vi "OpenQueryClose.vi"(8 "error in (no error)":errorcluster, 10 "timeout for receiving data [ms]":i32=5000, 11 "String to be sent":string="{\"id\":1234, \"command\":\"icl_info\"}") -> (0 "error out":errorcluster, 1 "contains error array?":bool, 2 "decoding error?":bool, 3 "Communicator out":refnum<class "Communicator.lvclass">, 5 "answer from device":string)   [LabVIEW 2023, in "GenericDevice.lvclass"]
uses:
  GenericDevice.lvclass
  Communicator/Communicator.lvclass
  GenericDevice.lvclass/GenericDevice.ctl
panel:
  # "Connector Pane"
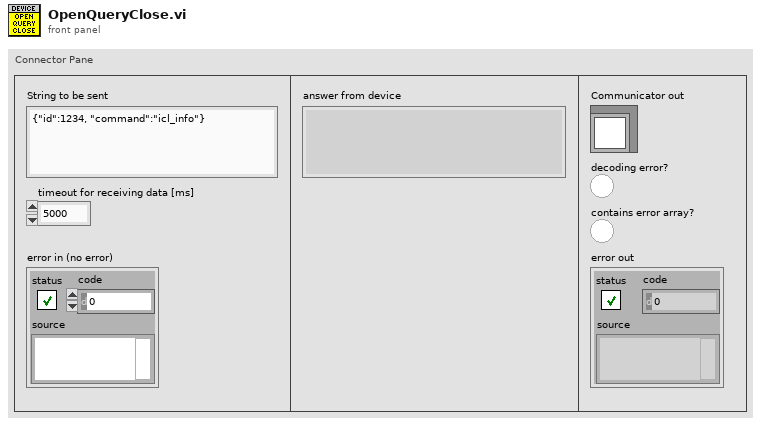
[diagram p1: front panel]
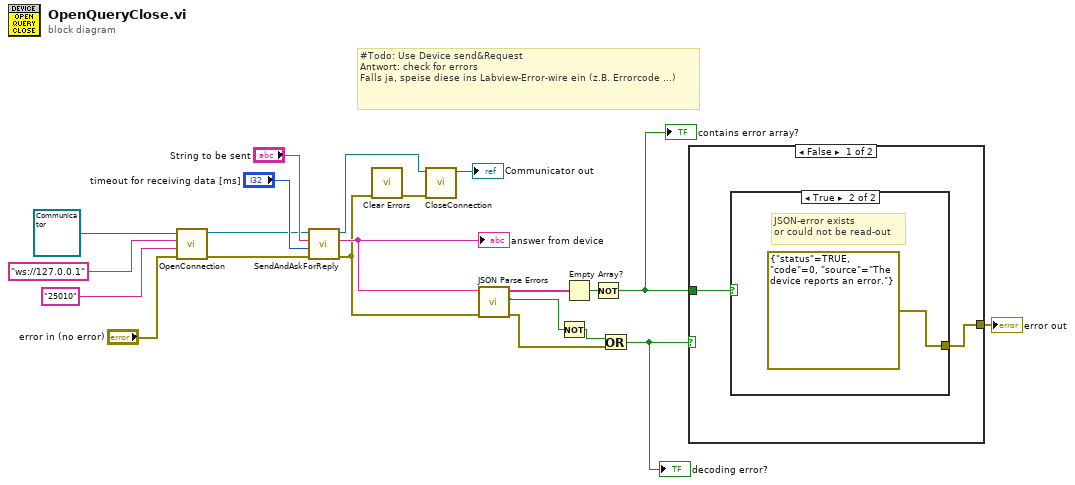
[diagram p0: block diagram]
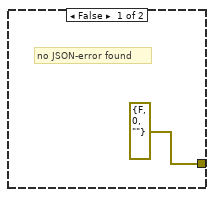
[diagram p2: hidden frame]
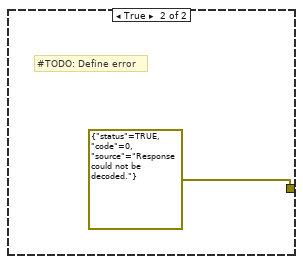
[diagram p3: hidden frame]
diagram:
  # "#Todo: Use Device send&Request\nAntwort: check for errors\nFalls ja, speise diese ins Labview-Error-wire ein (z.B. Errorcode ...)"
  n1 = call-dynamic "OpenConnection.vi"("error in (no error)"="error in (no error)", "WS Server Port"="25010", "WS Server IP"="ws://127.0.0.1", "Communicator in"=refnum<class "Communicator.lvclass"> refnum ("Communicator")) -> ("error out"=w10:errorcluster, "Communicator out"=w9:refnum<class "Communicator.lvclass">)  [unwired: 5 in, 1 out]
  n2 = call-dynamic "SendAndAskForReply.vi"("error in (no error)"=w10, "timeout for receiving data [ms]"="timeout for receiving data [ms]", "String to be sent"="String to be sent", "Communicator in"=w9) -> ("error out"=w1:errorcluster, "Data"=w2:string, "Communicator out"=w8:refnum<class "Communicator.lvclass">)  [unwired: 5 in]
  "answer from device" <- w2
  n3 = call <vilib>:"Clear Errors.vi"("error in (no error)"=w1) -> ("error out"=w4:errorcluster)  [unwired: 5 in, 1 out]
  n4 = call-dynamic "CloseConnection.vi"("error in (no error)"=w4, "Communicator in"=w8) -> ("Communicator out"=→"Communicator out":refnum<class "Communicator.lvclass">)  [unwired: 8 in, 1 out]
  n5 = call "JSON Parse Errors.vi"("error in (no error)"=w1, "JSON command"=w2) -> ("error out"=w6:errorcluster, "isErrorFree?"=w3:bool, "formatted error array"=w5:string[])  [unwired: 5 in, 2 out]
  n6 = Not(x=w3) -> (.not. x?=w18:bool)
  n7 = Empty Array?(array=w5) -> (empty?=w16:bool)
  n8 = Not(x=w16) -> (.not. x?=w15:bool)
  "contains error array?" <- w15
  n9 = Or(x=w18, y=w6) -> (x .or. y?=w17:bool)
  "decoding error?" <- w17
  n10 = case shown="False" w17 {
    tunnel: [w23 errorcluster {"status"=TRUE, "code"=0, "source"="Response could not be decoded."} ("error in (no error)")] -> w19
    tunnel: w15 -> [w22 _]
    frame False {
      n11 = case shown="True" w22 {
        tunnel: [errorcluster {"status"=FALSE, "code"=0, "source"=""} ("error in (no error)") errorcluster {"status"=TRUE, "code"=0, "source"="The device reports an error."} ("error in (no error)")] -> w23
        frame False {
          # "no JSON-error found"
        }
        frame True {
          # "JSON-error exists\nor could not be read-out"
        }
      }
    }
    frame True {
      # "#TODO: Define error"
    }
  }
  "error out" <- w19
